vi "Configure Modulation (Frequency-Shift Keying).vi"(0 "VISA resource name":refnum<visa-resource-name>, 1 "FSK Rate (10.00 Hz)":dbl=10.0 min=0.002 max=100000.0 format="%.2f", 2 "Hop Frequency (100.00 Hz)":dbl=100.0 min=1e-06 max=80000000.0 format="%.2f", 5 "Enable FSK Modulation (T: Enable)":bool=TRUE, 7 "FSK Modulation Source (0: Internal)":u16(ring) items=["Internal", "External"], 11 "error in (no error)":errorcluster) -> (4 "VISA resource name out":refnum<visa-resource-name>, 15 "error out":errorcluster)   [LabVIEW 2026, in "Agilent 33XXX Series.lvlib"]
doc: "Allows and configures Frequency-Shift Keying (FSK) modulation. The function generator shifts its output frequency between two present values. The carrier waveform shape and parameters are set by config waveform function.\n\nNote:\n(1) Before using this mode, all other modes must be turned off.\n(2) The carrier waveform shape and parameters are set by the Configure Standard Waveform vi.\n(3) This VI is not valid in 33210."
uses:
  Agilent 33XXX Series.lvlib
panel:
  # "Internal FSK Settings"
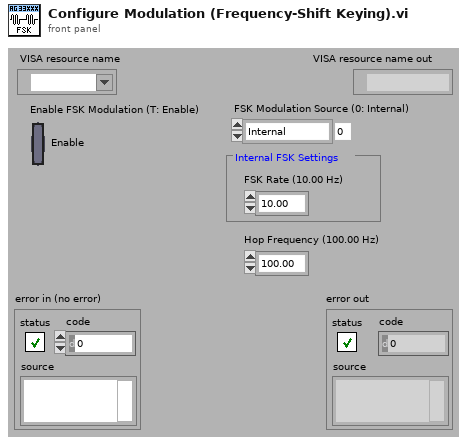
[diagram p1: front panel]
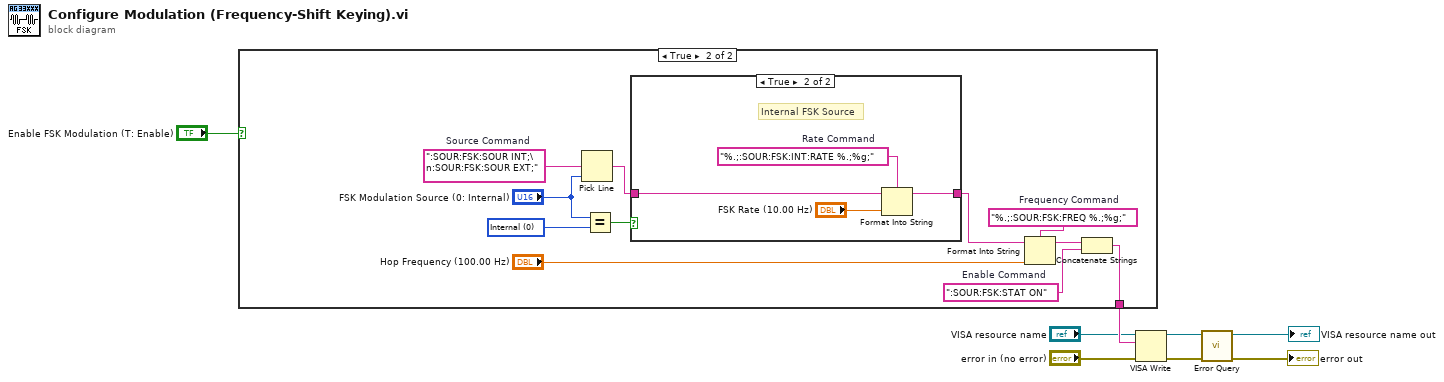
[diagram p0: block diagram]
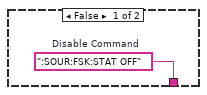
[diagram p2: hidden frame]
diagram:
  n1 = case shown="True" "Enable FSK Modulation (T: Enable)" {
    tunnel: [w9 w13] -> w8
    frame False {
      w9 = ":SOUR:FSK:STAT OFF"  # Disable Command
    }
    frame True {
      w12 = ":SOUR:FSK:STAT ON"  # Enable Command
      w17 = "%.;:SOUR:FSK:FREQ %.;%g;"  # Frequency Command
      w19 = u16 0 items=["Internal", "External"] ("Source (0: Internal)")
      w20 = ":SOUR:FSK:SOUR INT;\n:SOUR:FSK:SOUR EXT;"  # Source Command
      n2 = Pick Line(multi-line string=w20, line index="FSK Modulation Source (0: Internal)") -> (output string=w15:string)  [unwired: 1 in]
      n3 = Equal?(x="FSK Modulation Source (0: Internal)", y=w19) -> (x = y?=w18:bool)
      n4 = case shown="True" w18 {
        tunnel: w15 -> [w21 w22]
        tunnel: [w21 w24] -> w16
        frame False {
          # "External FSK Source"
        }
        frame True {
          w25 = "%.;:SOUR:FSK:INT:RATE %.;%g;"  # Rate Command
          # "Internal FSK Source"
          n5 = Format Into String(format string=w25, initial string=w22, "FSK Rate (10.00 Hz)") -> (resulting string=w24:string)  [unwired: 1 in, 1 out]
        }
      }
      n6 = Format Into String(format string=w17, initial string=w16, "Hop Frequency (100.00 Hz)") -> (resulting string=w14:string)  [unwired: 1 in, 1 out]
      n7 = Concatenate Strings(w14, w12) -> (w13:string)
    }
  }
  n8 = VISA Write(VISA resource name="VISA resource name", write buffer=w8, error in (no error)="error in (no error)") -> (VISA resource name out=w7:refnum<visa-resource-name>, error out=w6:errorcluster)  [unwired: 1 out]
  n9 = call "Error Query.vi"("error in (no error)"=w6, "VISA resource name"=w7) -> ("error out"=→"error out":errorcluster, "VISA resource name out"=→"VISA resource name out":refnum<visa-resource-name>)  [unwired: 6 in, 2 out]
